vi "Application Settings.vi"(8 "error in":errorcluster, 11 "Controller in":refnum<class "Controller.lvclass">) -> (0 "error out":errorcluster, 3 "Controller out":refnum<class "Controller.lvclass">)   [LabVIEW 2021, in "Controller.lvlib" / "Controller.lvclass"]
uses:
  Controller.lvclass
  Controller.lvclass/Controller.ctl
  UserInterface/UserInterface Messages/Log Data Msg/Log Data Msg.lvclass/Log Data Msg.ctl
  <vilib>/ActorFramework/Message Enqueuer/Message Enqueuer.lvclass/Message Enqueuer.ctl
  PLCHandler/PLCHandler Messages/Init Msg/Init Msg.lvclass/Init Msg.ctl
  <vilib>/ActorFramework/Message Enqueuer/Enqueue.vi
  UserInterface/UserInterface Messages/Log Data Msg/Log Data Msg.lvclass
  C:/Program Files/National Instruments/LabVIEW 2021/vi.lib/ActorFramework/Message/Message.lvclass
  PLCHandler/PLCHandler Messages/DeInit Msg/DeInit Msg.lvclass
  PLCHandler/PLCHandler Messages/Init Msg/Init Msg.lvclass
  <vilib>/ActorFramework/Message Priority Queue/Priority Enqueue.vi
panel:
  in  "Cancel":bool
  in  "Save":bool
  in  "Settings Tab":enum32{"Application Settings.."}(tab)
  in  "Total Img Read Address":u32
  in  "Acknowledge Address":u16=2110
  in  "Acquisition Address":u16=2108
  in  "Wakeup Address":u16=2112
  in  "Baud Rate":u32=9600
  in  "Enabled?":bool
  in  "Secondary Path":path
  in  "Primary Path":path
  in  "PLC Port":refnum<visa-resource-name>
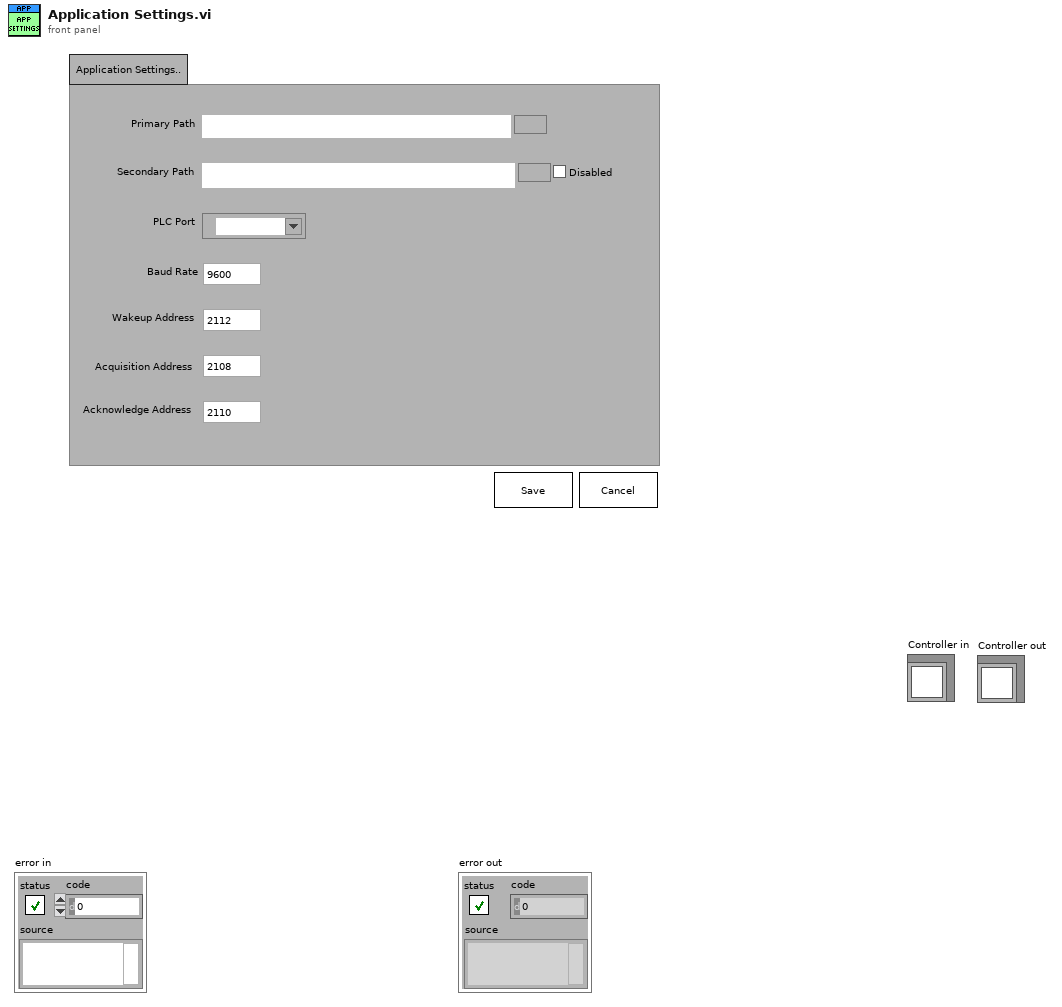
[diagram p1: front panel]
types:
  T1 = enum16{"Poll", "Intialize", "Save Settings", "Error", "Exit"}
  T2 = typedef "Storage Settings.ctl" = cluster{"Primary Path":path, "Backup Storage?":bool, "Backup Path":path, "Component Name Prefix":string, "Image Format":T3}
  T3 = typedef "Image Formats.ctl" = enum16{"<Select>", "TIFF", "RAW"}
  T4 = typedef "PLC Settings.ctl" = cluster{"Port":refnum<visa-resource-name>, "BaudRate":u32, "Wakeup Signal Address ":u16, "Acquisiton Address":u16, "Acknowledgement Address":u16, "Sleep Address":u32}
  T5 = cluster{"Storage Settings":T2, "PLC Settings":T4, "Total Images":u32}
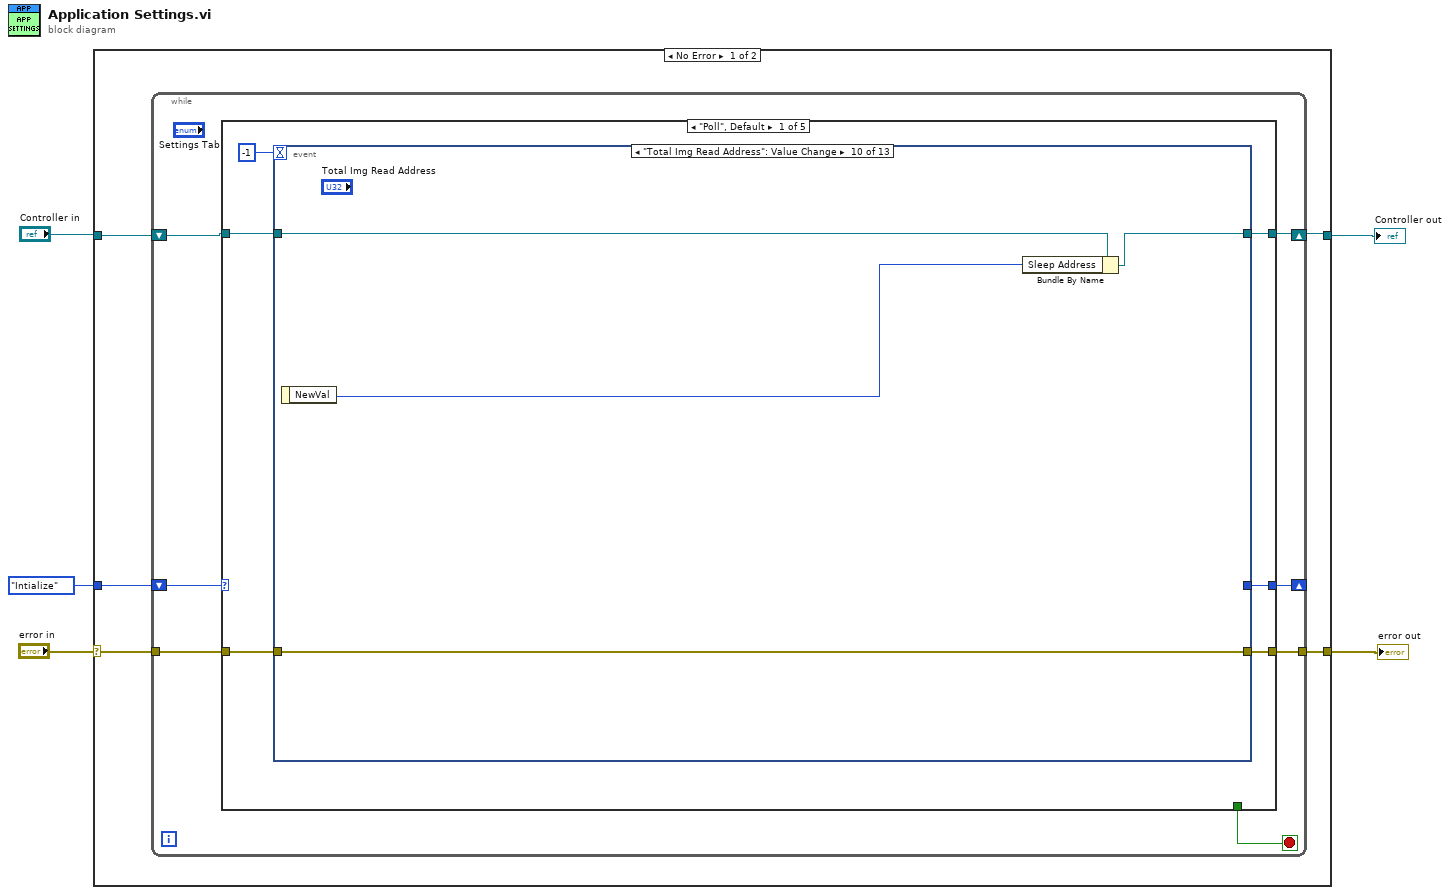
[diagram p0: block diagram]
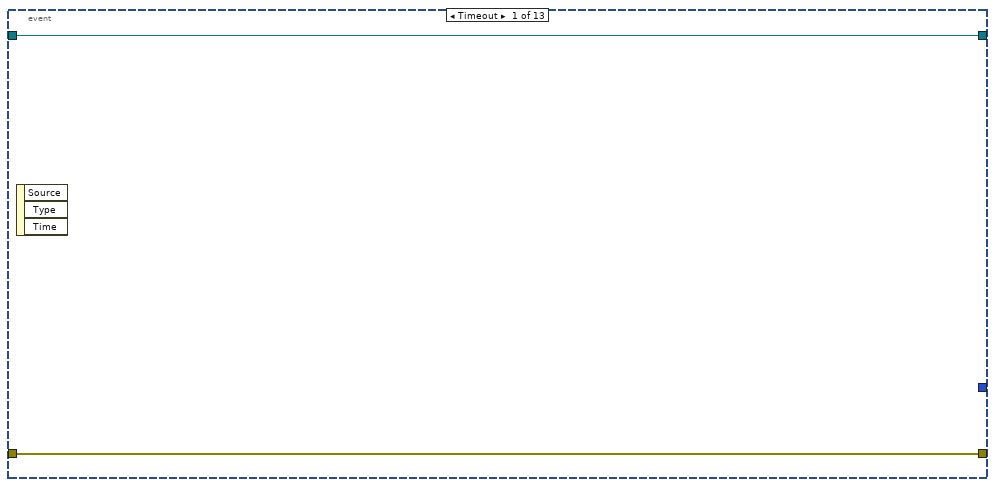
[diagram p2: hidden frame]
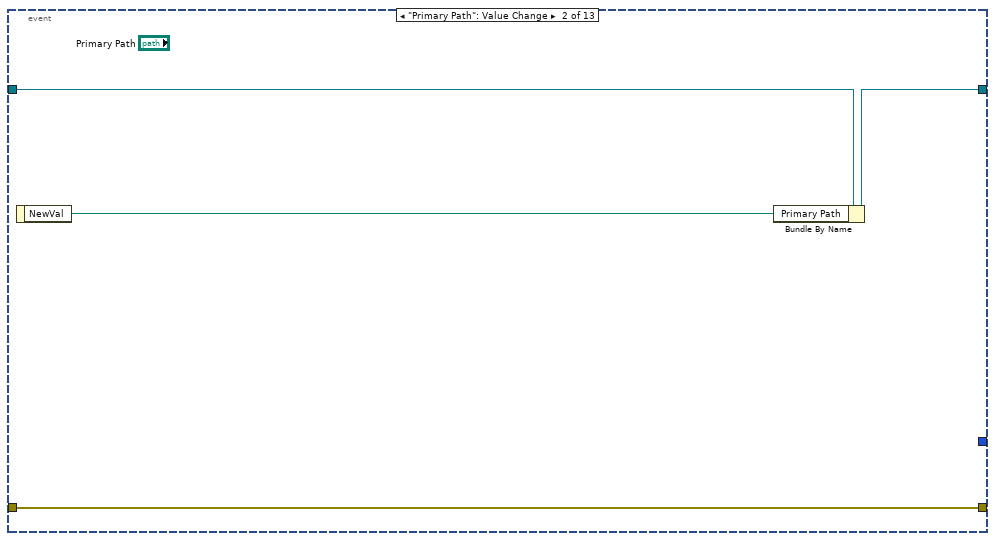
[diagram p3: hidden frame]
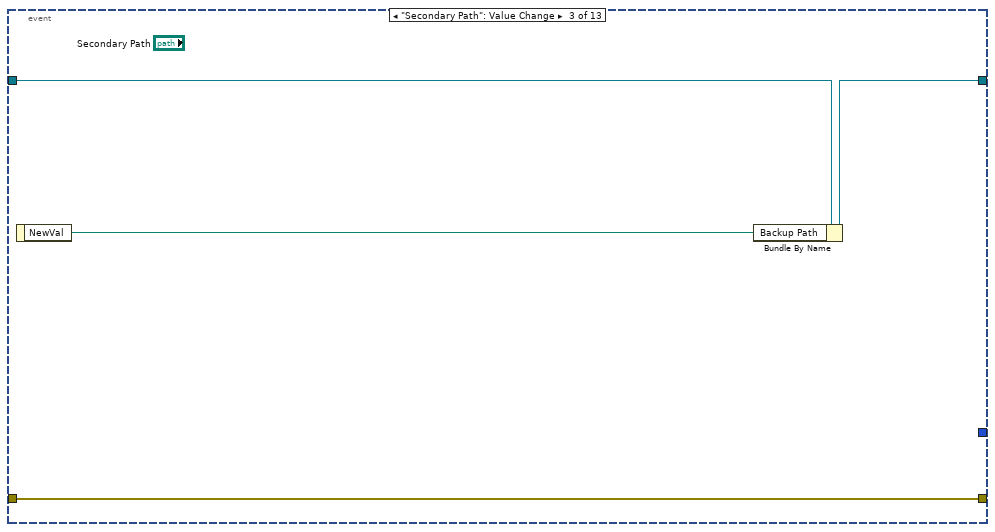
[diagram p4: hidden frame]
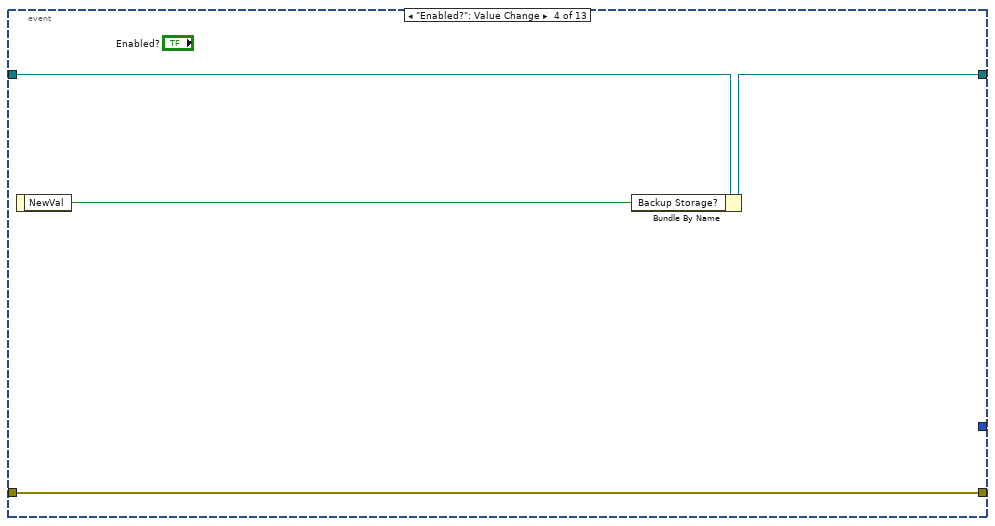
[diagram p5: hidden frame]
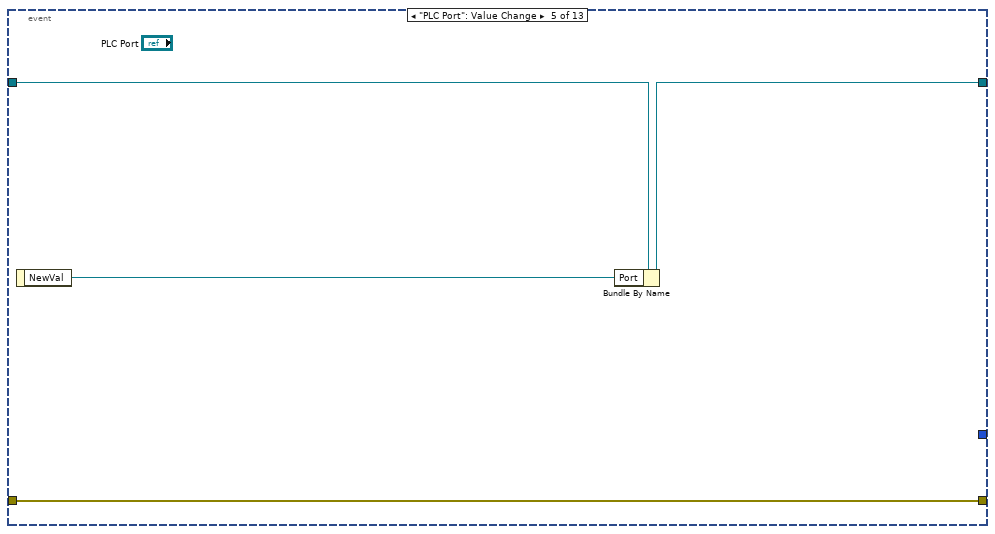
[diagram p6: hidden frame]
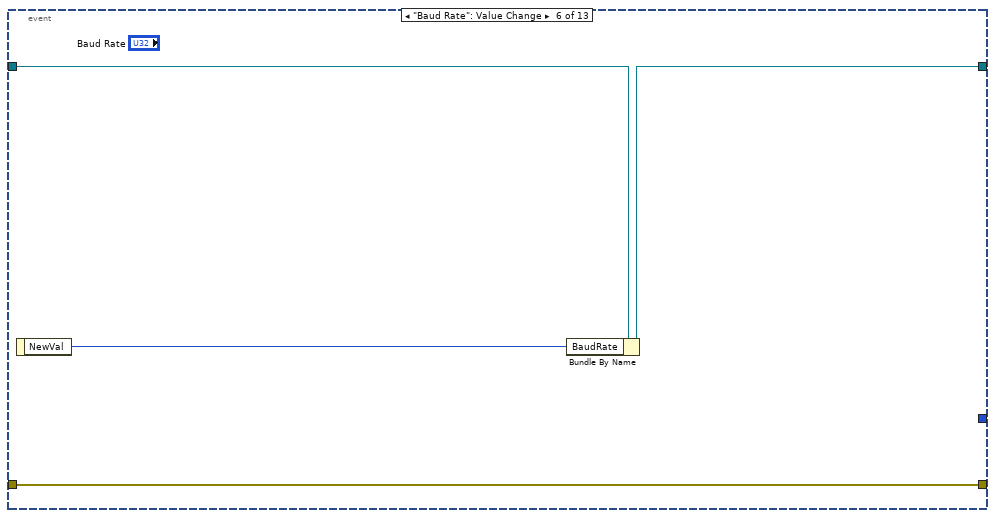
[diagram p7: hidden frame]
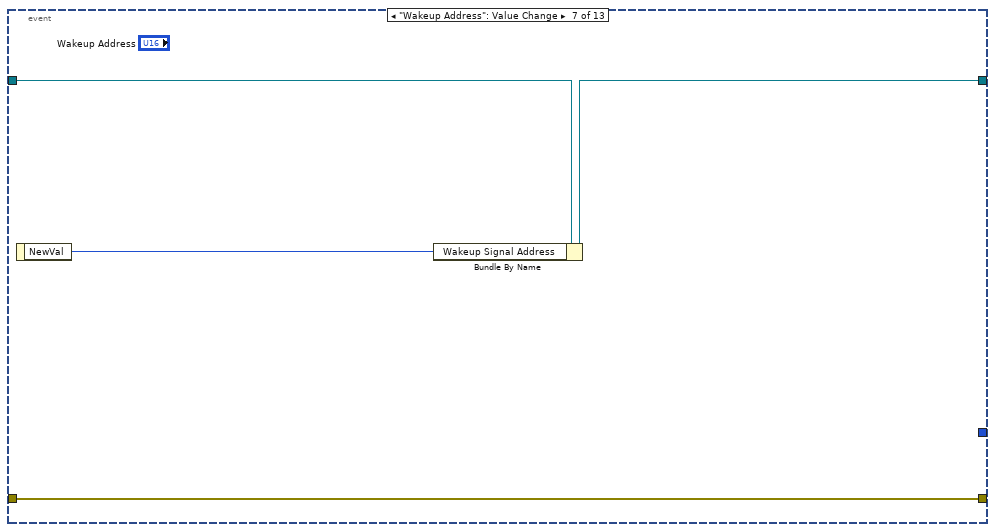
[diagram p8: hidden frame]
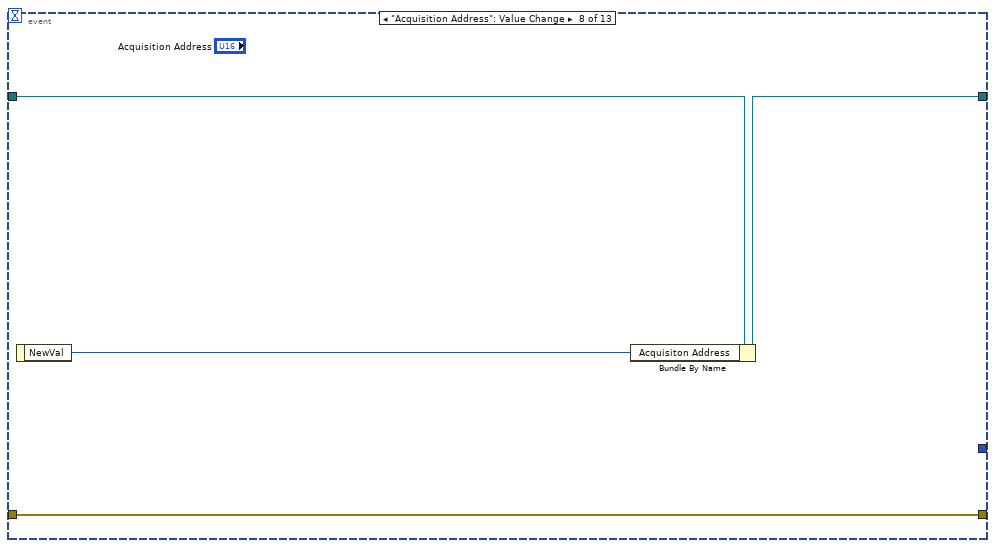
[diagram p9: hidden frame]
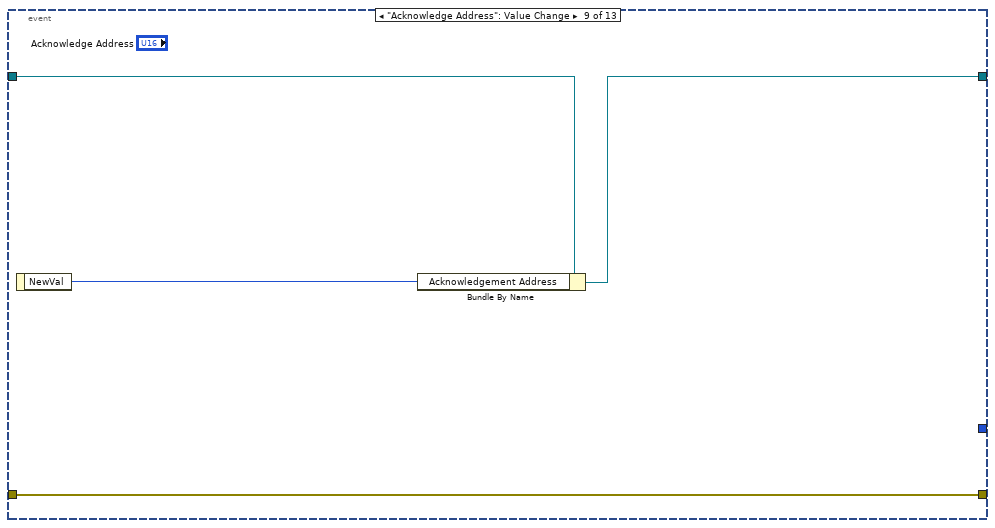
[diagram p10: hidden frame]
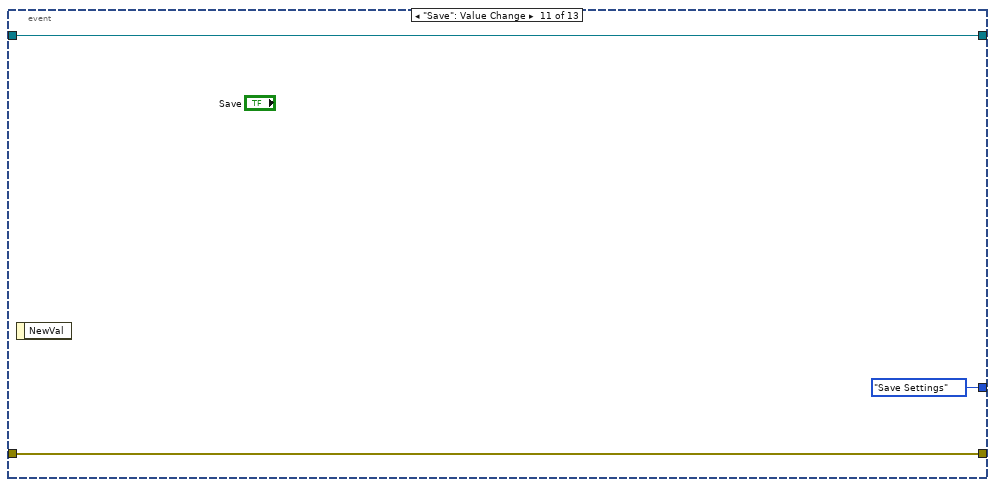
[diagram p11: hidden frame]
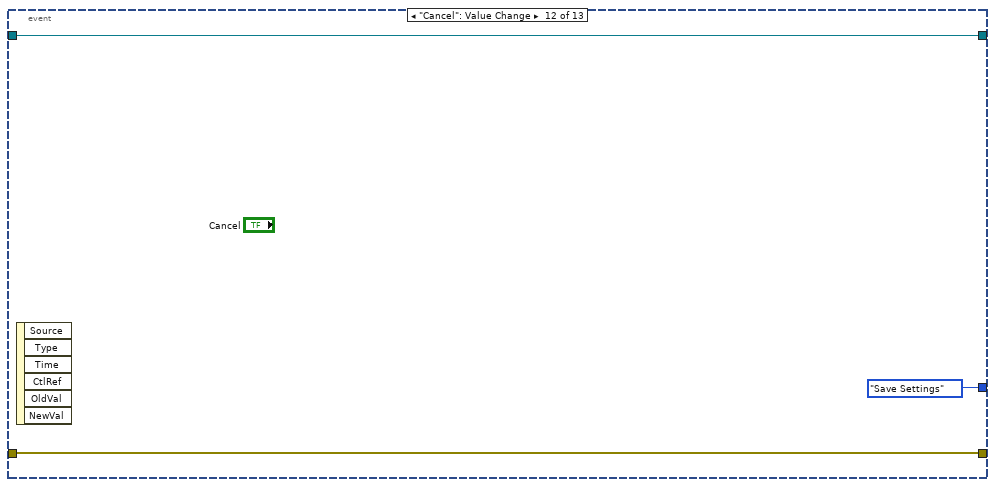
[diagram p12: hidden frame]
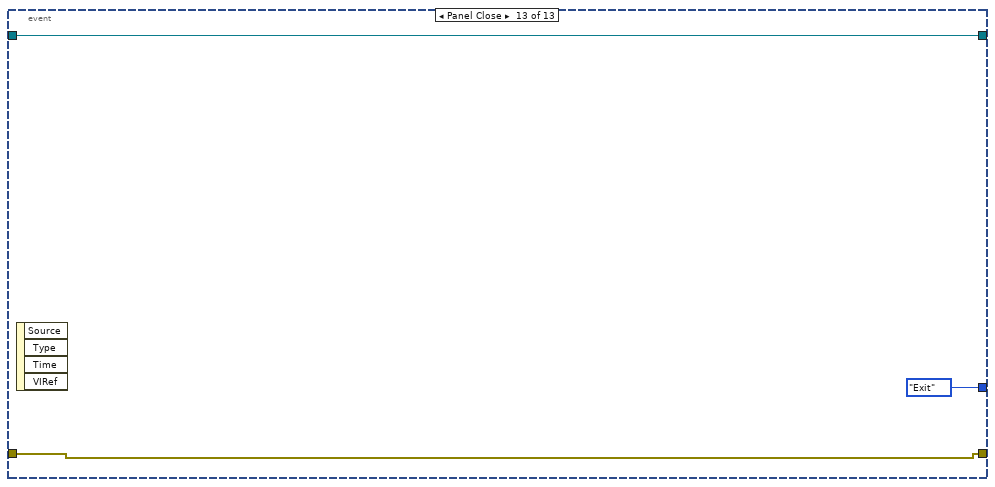
[diagram p13: hidden frame]
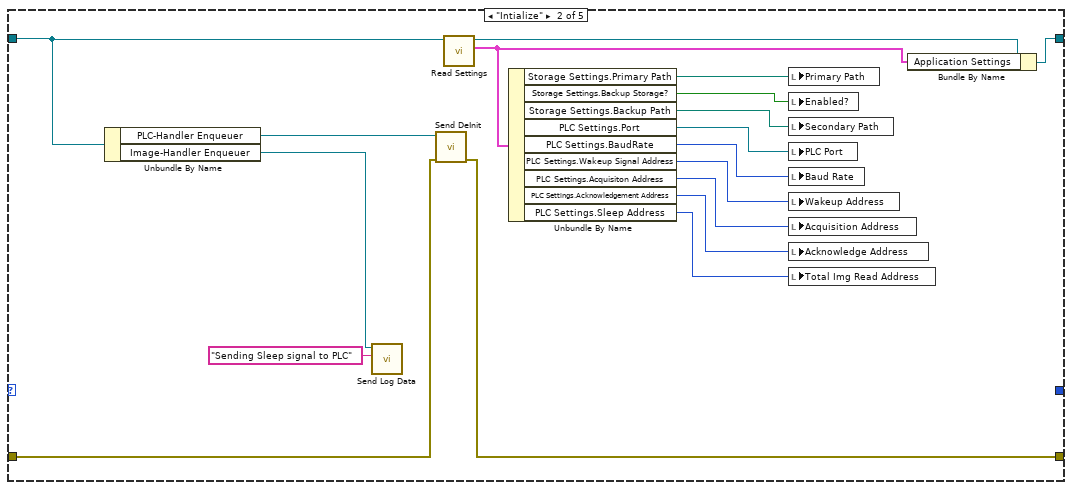
[diagram p14: hidden frame]
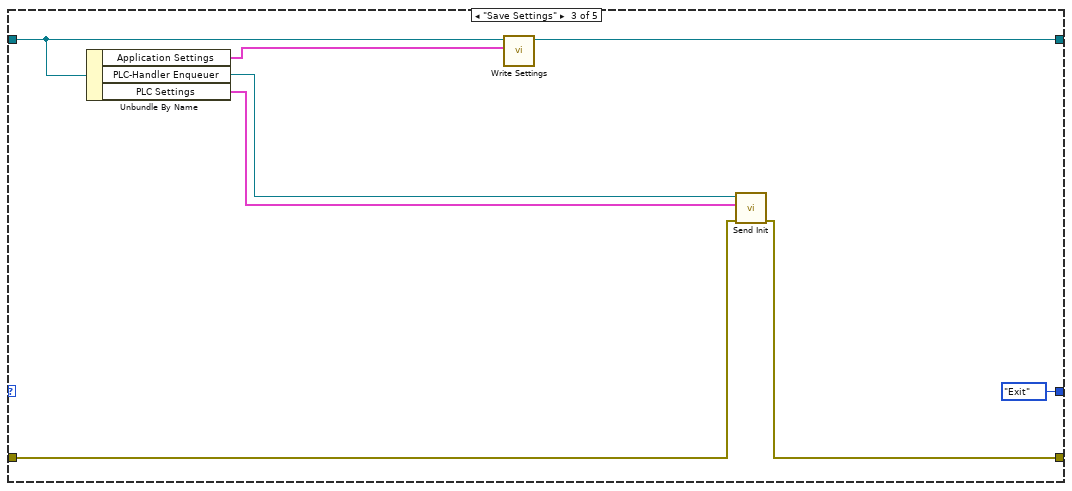
[diagram p15: hidden frame]
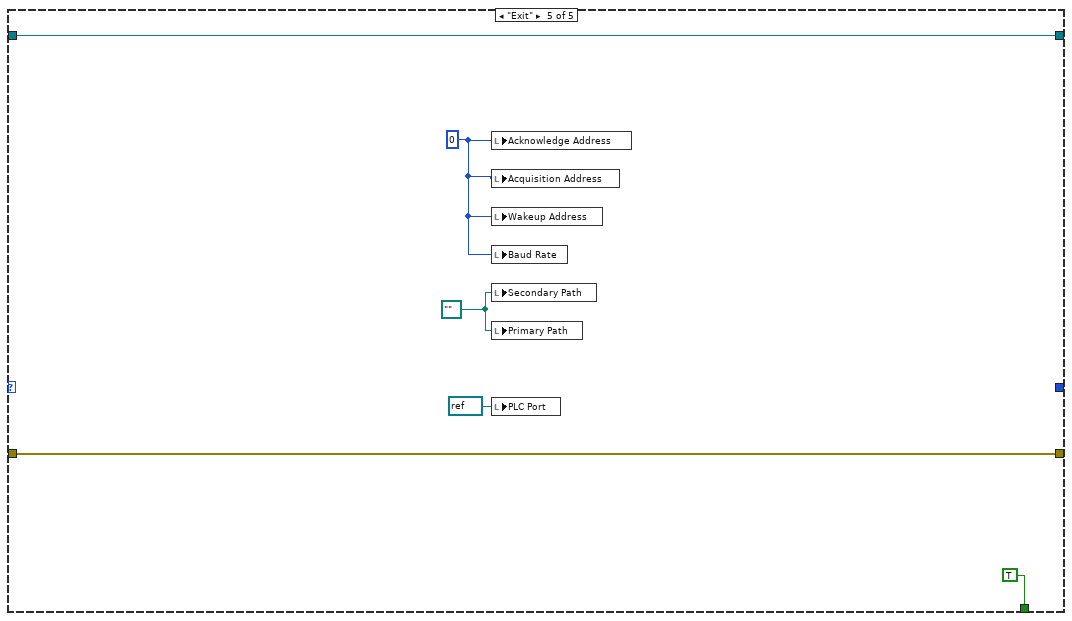
[diagram p17: hidden frame]
diagram:
  n1 = case shown="No Error" "error in" {
    selector: "error in" -> [w7 w106]
    tunnel: [w6 w106] -> w4
    tunnel: [w9 w105] -> w3
    tunnel: "Controller in" -> [w10 w105]
    tunnel: T1."Intialize" -> [w8 _]
    frame No Error {
      n2 = while {
        shift-right: [w14] -> _
        shift-left: w8 -> [w15]
        tunnel: w7 -> [w13]
        tunnel: [w12] -> w6
        shift-right: [w16] -> w9
        shift-left: w10 -> [w17]
        stop <- w11 stop-if-true
        n3 = case shown="\"Poll\", Default" w15 {
          tunnel: w17 -> [w23 w84 w91 w97 w102]
          tunnel: [w22 w88 w90 w97 w102] -> w16
          tunnel: [w20 _ T1."Exit" _ _] -> w14
          tunnel: w13 -> [w19 w86 w93 w98 w103]
          tunnel: [w18 w85 w94 w98 w103] -> w12
          tunnel: [_ _ _ _ TRUE] -> w11
          frame "Poll", Default {
            n4 = event shown="[9] \"Total Img Read Address\": Value Change" {
              selector: _ -> [_ _ _ _ _ _ _ _ _ _ _ _ _]
              dyn-events: _ -> [_ _ _ _ _ _ _ _ _ _ _ _ _]
              timeout: -1 -> [_ _ _ _ _ _ _ _ _ _ _ _ _]
              tunnel: [_ _ _ _ _ _ _ _ _ _ T1."Save Settings" T1."Save Settings" T1."Exit"] -> w20
              tunnel: w23 -> [w25 w29 w33 w37 w41 w45 w49 w53 w57 w60 w63 w65 w68]
              tunnel: [w25 w27 w31 w35 w39 w43 w47 w51 w55 w59 w63 w65 w68] -> w22
              tunnel: w19 -> [w24 w28 w32 w36 w40 w44 w48 w52 w56 w61 w62 w66 w69]
              tunnel: [w24 w28 w32 w36 w40 w44 w48 w52 w56 w61 w62 w66 w69] -> w18
              event Timeout {
                n5 = event-data() -> ()  [unwired: 1 in, 3 out]
              }
              event "Primary Path": Value Change {
                n6 = event-data() -> ("NewVal"=w26:path)  [unwired: 1 in]
                n7 = Bundle By Name(cluster=w29, "Primary Path"=w26) -> (w27:refnum<class "Controller.lvclass">)
              }
              event "Secondary Path": Value Change {
                n8 = event-data() -> ("NewVal"=w30:path)  [unwired: 1 in]
                n9 = Bundle By Name(cluster=w33, "Backup Path"=w30) -> (w31:refnum<class "Controller.lvclass">)
              }
              event "Enabled?": Value Change {
                n10 = event-data() -> ("NewVal"=w34:bool)  [unwired: 1 in]
                n11 = Bundle By Name(cluster=w37, "Backup Storage?"=w34) -> (w35:refnum<class "Controller.lvclass">)
              }
              event "PLC Port": Value Change {
                n12 = event-data() -> ("NewVal"=w38:refnum<visa-resource-name>)  [unwired: 1 in]
                n13 = Bundle By Name(cluster=w41, "Port"=w38) -> (w39:refnum<class "Controller.lvclass">)
              }
              event "Baud Rate": Value Change {
                n14 = event-data() -> ("NewVal"=w42:u32)  [unwired: 1 in]
                n15 = Bundle By Name(cluster=w45, "BaudRate"=w42) -> (w43:refnum<class "Controller.lvclass">)
              }
              event "Wakeup Address": Value Change {
                n16 = event-data() -> ("NewVal"=w46:u16)  [unwired: 1 in]
                n17 = Bundle By Name(cluster=w49, "Wakeup Signal Address"=w46) -> (w47:refnum<class "Controller.lvclass">)
              }
              event "Acquisition Address": Value Change {
                n18 = event-data() -> ("NewVal"=w50:u16)  [unwired: 1 in]
                n19 = Bundle By Name(cluster=w53, "Acquisiton Address"=w50) -> (w51:refnum<class "Controller.lvclass">)
              }
              event "Acknowledge Address": Value Change {
                n20 = event-data() -> ("NewVal"=w54:u16)  [unwired: 1 in]
                n21 = Bundle By Name(cluster=w57, "Acknowledgement Address"=w54) -> (w55:refnum<class "Controller.lvclass">)
              }
              event "Total Img Read Address": Value Change {
                n22 = event-data() -> ("NewVal"=w58:u32)  [unwired: 1 in]
                n23 = Bundle By Name(cluster=w60, "Sleep Address"=w58) -> (w59:refnum<class "Controller.lvclass">)
              }
              event "Save": Value Change {
                n24 = event-data() -> ()  [unwired: 1 in, 1 out]
              }
              event "Cancel": Value Change {
                n25 = event-data() -> ()  [unwired: 1 in, 6 out]
              }
              event Panel Close {
                n26 = event-data() -> ()  [unwired: 1 in, 4 out]
              }
            }
          }
          frame "Intialize" {
            n27 = Unbundle By Name(w84) -> ("PLC-Handler Enqueuer"=w87:refnum<class "Message Enqueuer.lvclass">, "Image-Handler Enqueuer"=w82:refnum<class "Message Enqueuer.lvclass">)
            n28 = call "Send Log Data.vi"("Message"="Sending Sleep signal to PLC", "Message Enqueuer"=w82) -> ()  [unwired: 8 in, 2 out]
            n29 = call "Send DeInit.vi"("error in (no error)"=w86, "Message Enqueuer"=w87) -> ("error out"=w85:errorcluster)  [unwired: 8 in, 1 out]
            n30 = call "Read Settings.vi"("Controller in"=w84) -> ("App Settings"=w80:T5, "Controller out"=w83:refnum<class "Controller.lvclass">)  [unwired: 8 in, 1 out]
            n31 = Unbundle By Name(w80) -> ("Storage Settings.Primary Path"=w79:path, "Storage Settings.Backup Storage?"=w78:bool, "Storage Settings.Backup Path"=w77:path, "PLC Settings.Port"=w76:refnum<visa-resource-name>, "PLC Settings.BaudRate"=w75:u32, "PLC Settings.Wakeup Signal Address"=w74:u16, "PLC Settings.Acquisiton Address"=w73:u16, "PLC Settings.Acknowledgement Address"=w72:u16, "PLC Settings.Sleep Address"=w71:u32)
            n32 = local write "Primary Path"(w79) -> ()
            n33 = local write "Enabled?"(w78) -> ()
            n34 = local write "Secondary Path"(w77) -> ()
            n35 = local write "PLC Port"(w76) -> ()
            n36 = local write "Baud Rate"(w75) -> ()
            n37 = local write "Wakeup Address"(w74) -> ()
            n38 = local write "Acquisition Address"(w73) -> ()
            n39 = local write "Acknowledge Address"(w72) -> ()
            n40 = local write "Total Img Read Address"(w71) -> ()
            n41 = Bundle By Name(cluster=w83, "Application Settings"=w80) -> (w88:refnum<class "Controller.lvclass">)
          }
          frame "Save Settings" {
            n42 = Unbundle By Name(w91) -> ("Application Settings"=w89:T5, "PLC-Handler Enqueuer"=w92:refnum<class "Message Enqueuer.lvclass">, "PLC Settings"=w95:T4)
            n43 = call "Write Settings.vi"("App Settings"=w89, "Controller in"=w91) -> ("Controller out"=w90:refnum<class "Controller.lvclass">)  [unwired: 8 in, 1 out]
            n44 = call "Send Init.vi"("error in (no error)"=w93, "PLC Settings"=w95, "Message Enqueuer"=w92) -> ("error out"=w94:errorcluster)  [unwired: 7 in, 1 out]
          }
          frame "Error" {
          }
          frame "Exit" {
            w100 = path "" ("Primary Path")
            w101 = 0
            n45 = local write "Acknowledge Address"(w101) -> ()
            n46 = local write "Acquisition Address"(w101) -> ()
            n47 = local write "Wakeup Address"(w101) -> ()
            n48 = local write "Baud Rate"(w101) -> ()
            n49 = local write "Secondary Path"(w100) -> ()
            n50 = local write "Primary Path"(w100) -> ()
            n51 = local write "PLC Port"(refnum<visa-resource-name> refnum ("PLC Port")) -> ()
          }
        }
      }
    }
    frame Error {
    }
  }
  "error out" <- w4
  "Controller out" <- w3
